vi "Main.vi"() -> ()   [LabVIEW 2017]
doc: "This Continuous Measurement sample project is based on the Queued Message Handler template.\n\nThe Event Handling Loop generates messages based on user interface actions.\n\nThe Message Handling Loop processes messages generated by the Event Handling Loop, or by other messages. There are also Acquisition and Logging message handling loop subVIs, and a chart updating loop."
uses:
  controls/UI Data.ctl
  support/libs/PMU Buffer/Buffer DATA cluster.ctl
  controls/UI State.ctl
  acquisition/Acquisition Settings.ctl
  acquisition/Acquisition State.ctl
  logging/Logging Configuration.ctl
  logging/Logging State.ctl
  support/libs/PMU Buffer/Buffer Settings.ctl
  processing/Processing Settings.ctl
  controls/Acquired Data.ctl
  <vilib>/Utility/error.llb/DialogType.ctl
  support/libs/PMU Buffer/Buffer state.ctl
  b850246f-c621-4cc8-8cdb-6c63488b8d16.vi
  d6c7b380-5ef8-42a0-a533-ce26cb609579.vi
  5953c9e4-e6ed-48ce-a3e3-f4074e595e54.vi
  308fbb3a-e3c1-4651-8528-14e79cd65b6c.vi
  e1cf4c14-b580-4597-8acf-5221adc64a8a.vi
  17f702fa-b3ef-4227-89b6-1808d4fdff79.vi
  support/Message Queue/Enqueue Message (Single).vi
  <vilib>/S3DK/PMU Recorder Light/PRL Channel Selector.vi
  support/settings/Get Config File Path.vi
  <vilib>/Utility/xml.llb/Read From XML File.vi
  <vilib>/Utility/xml.llb/Read From XML File(string).vi
  <vilib>/Utility/xml.llb/Write to XML File.vi
  <vilib>/Utility/xml.llb/Write to XML File(string).vi
  <vilib>/Utility/error.llb/Error Cluster From Error Code.vi
  <vilib>/ErrorRing/Error Ring.xnode
  acquisition/Acquisition.lvlib
  logging/Logging.lvlib
  support/User Event - Stop/User Event - Stop.lvlib
  support/Message Queue/Message Queue.lvlib
  support/settings/Settings Dialog.vi
  support/settings/Settings.lvlib
  processing/Processing.lvlib
  support/libs/PMU Buffer/PMU data buffer.lvlib
  <vilib>/S3DK/PMU Recorder Light/PMU Recorder Light.lvlib
panel:
  in  "Data Selector":bool
  in  "PRL Visible":bool
  out "Buffer Active":bool
  out "Config File":bool
  out "Connected":bool
  out "Error":bool
  out "Processing":bool=TRUE
  out "Display":bool
  out "Acquisition":bool=TRUE
  out "Events":bool=TRUE
  out "Buffer":bool
  out "UI Control":bool
  out "Waveform Chart":dbl[](graph)
  in  "Settings":bool
  in  "Start":bool
  in  "Stop":bool
  out "Status":string
  in  "Exit":bool
  # "Continuous Measurement Data Logger"
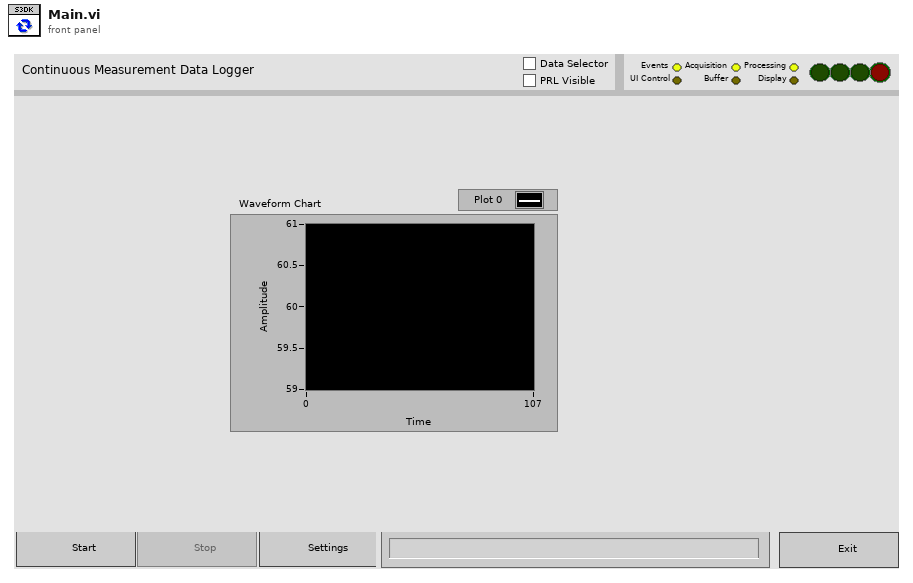
[diagram p1: front panel]
types:
  T1 = cluster{"Acq":refnum<notifier>, "Log":refnum<notifier>, "Proc":refnum<notifier>}
  T2 = typedef "Acquired Data.ctl" = cluster{"Data":dbl[]}
  T3 = typedef "Processing.lvlib/Processing Settings.ctl" = cluster{"Settings":string, "Parameters":T4, "Refresh Rate":u32}
  T4 = typedef "PMU data buffer.lvlib/Buffer Settings.ctl" = cluster{"Index":i32, "Size":i32, "Samples":i32, "Ordered ?":bool}
  T5 = typedef "Logging.lvlib/Logging Configuration.ctl" = cluster{"Logging State":T6, "Settings":string, "Buffer":T4}
  T6 = typedef "Logging.lvlib/Logging State.ctl" = enum16{"Idle", "Logging"}
  T7 = typedef "Acquisition.lvlib/Acquisition Settings.ctl" = cluster{"State":T8, "Settings":string, "Online":bool, "S3DK":cluster{"Signals":cluster{"Phasor":string[], "Analog":string[], "Digital":string[]}}, "CSV":cluster{"CSV Path":path, "Index":i32, "Parcel Length":i32, "EOF?":bool}}
  T8 = typedef "Acquisition.lvlib/Acquisition State.ctl" = enum16{"Idle", "Idle S3DK", "Acquiring S3DK", "Idle CSV", "Acquiring CSV"}
  T9 = typedef "UI State.ctl" = enum16{"Idle", "Acquiring and Logging", "Waiting for Exit", "Waiting for Exit (Acq Stopped)", "Waiting for Exit (Log Stopped)", "Waiting for Stop", "Waiting for Stop (Acq Stopped)", "Waiting for Stop (Log Stopped)"}
  T10 = typedef "PMU data buffer.lvlib/Buffer DATA cluster.ctl" = cluster{timestamp, csg[], sgl[]}
  T11 = typedef "UI Data.ctl" = cluster{"Start Ref":refnum<vi>, "Stop Ref":refnum<vi>, "Settings Ref":refnum<vi>, "Exit Ref":refnum<vi>, "Status Ref":refnum<vi>, "Data Ref":refnum<vi>, "Data Selector":refnum<vi>, "PRL Visible":refnum<vi>}
  T12 = typedef "Message Queue.lvlib/All Message Queues.ctl" = cluster{"UI":refnum<queue>, "Acquisition":refnum<queue>, "Logging":refnum<queue>, "Processing":refnum<queue>}
  T13 = enum16{"Run", "Startup", "Get Status", "Pause", "Continue", "Shutdown", "Abort", "Open Panel", "Close Panel"}
  T14 = typedef "DialogType.ctl" = u16
  T15 = enum32{"Invalid", "Standard", "Closed", "Hidden", "Minimized", "Maximized"}
  T16 = cluster{"Data Cluster":T7, "Logging Configuration":T5, "Processing Settings":T3}
  T17 = typedef "Settings.lvlib/Settings.ctl" = cluster{"Acquisition":T7, "Logging":T5, "Processing":T3}
  T18 = typedef "PMU data buffer.lvlib/Buffer state.ctl" = enum16{"Init", "Change Size", "Flush", "Exit", "Add", "Get", "Hist_Toggle", "Add_Serv"}
  T19 = typedef "PMU data buffer.lvlib/Buffer DATA OUT ordered.ctl" = cluster{"Timestamp":timestamp[], "Phasor":csg[][], "Analog":sgl[][]}
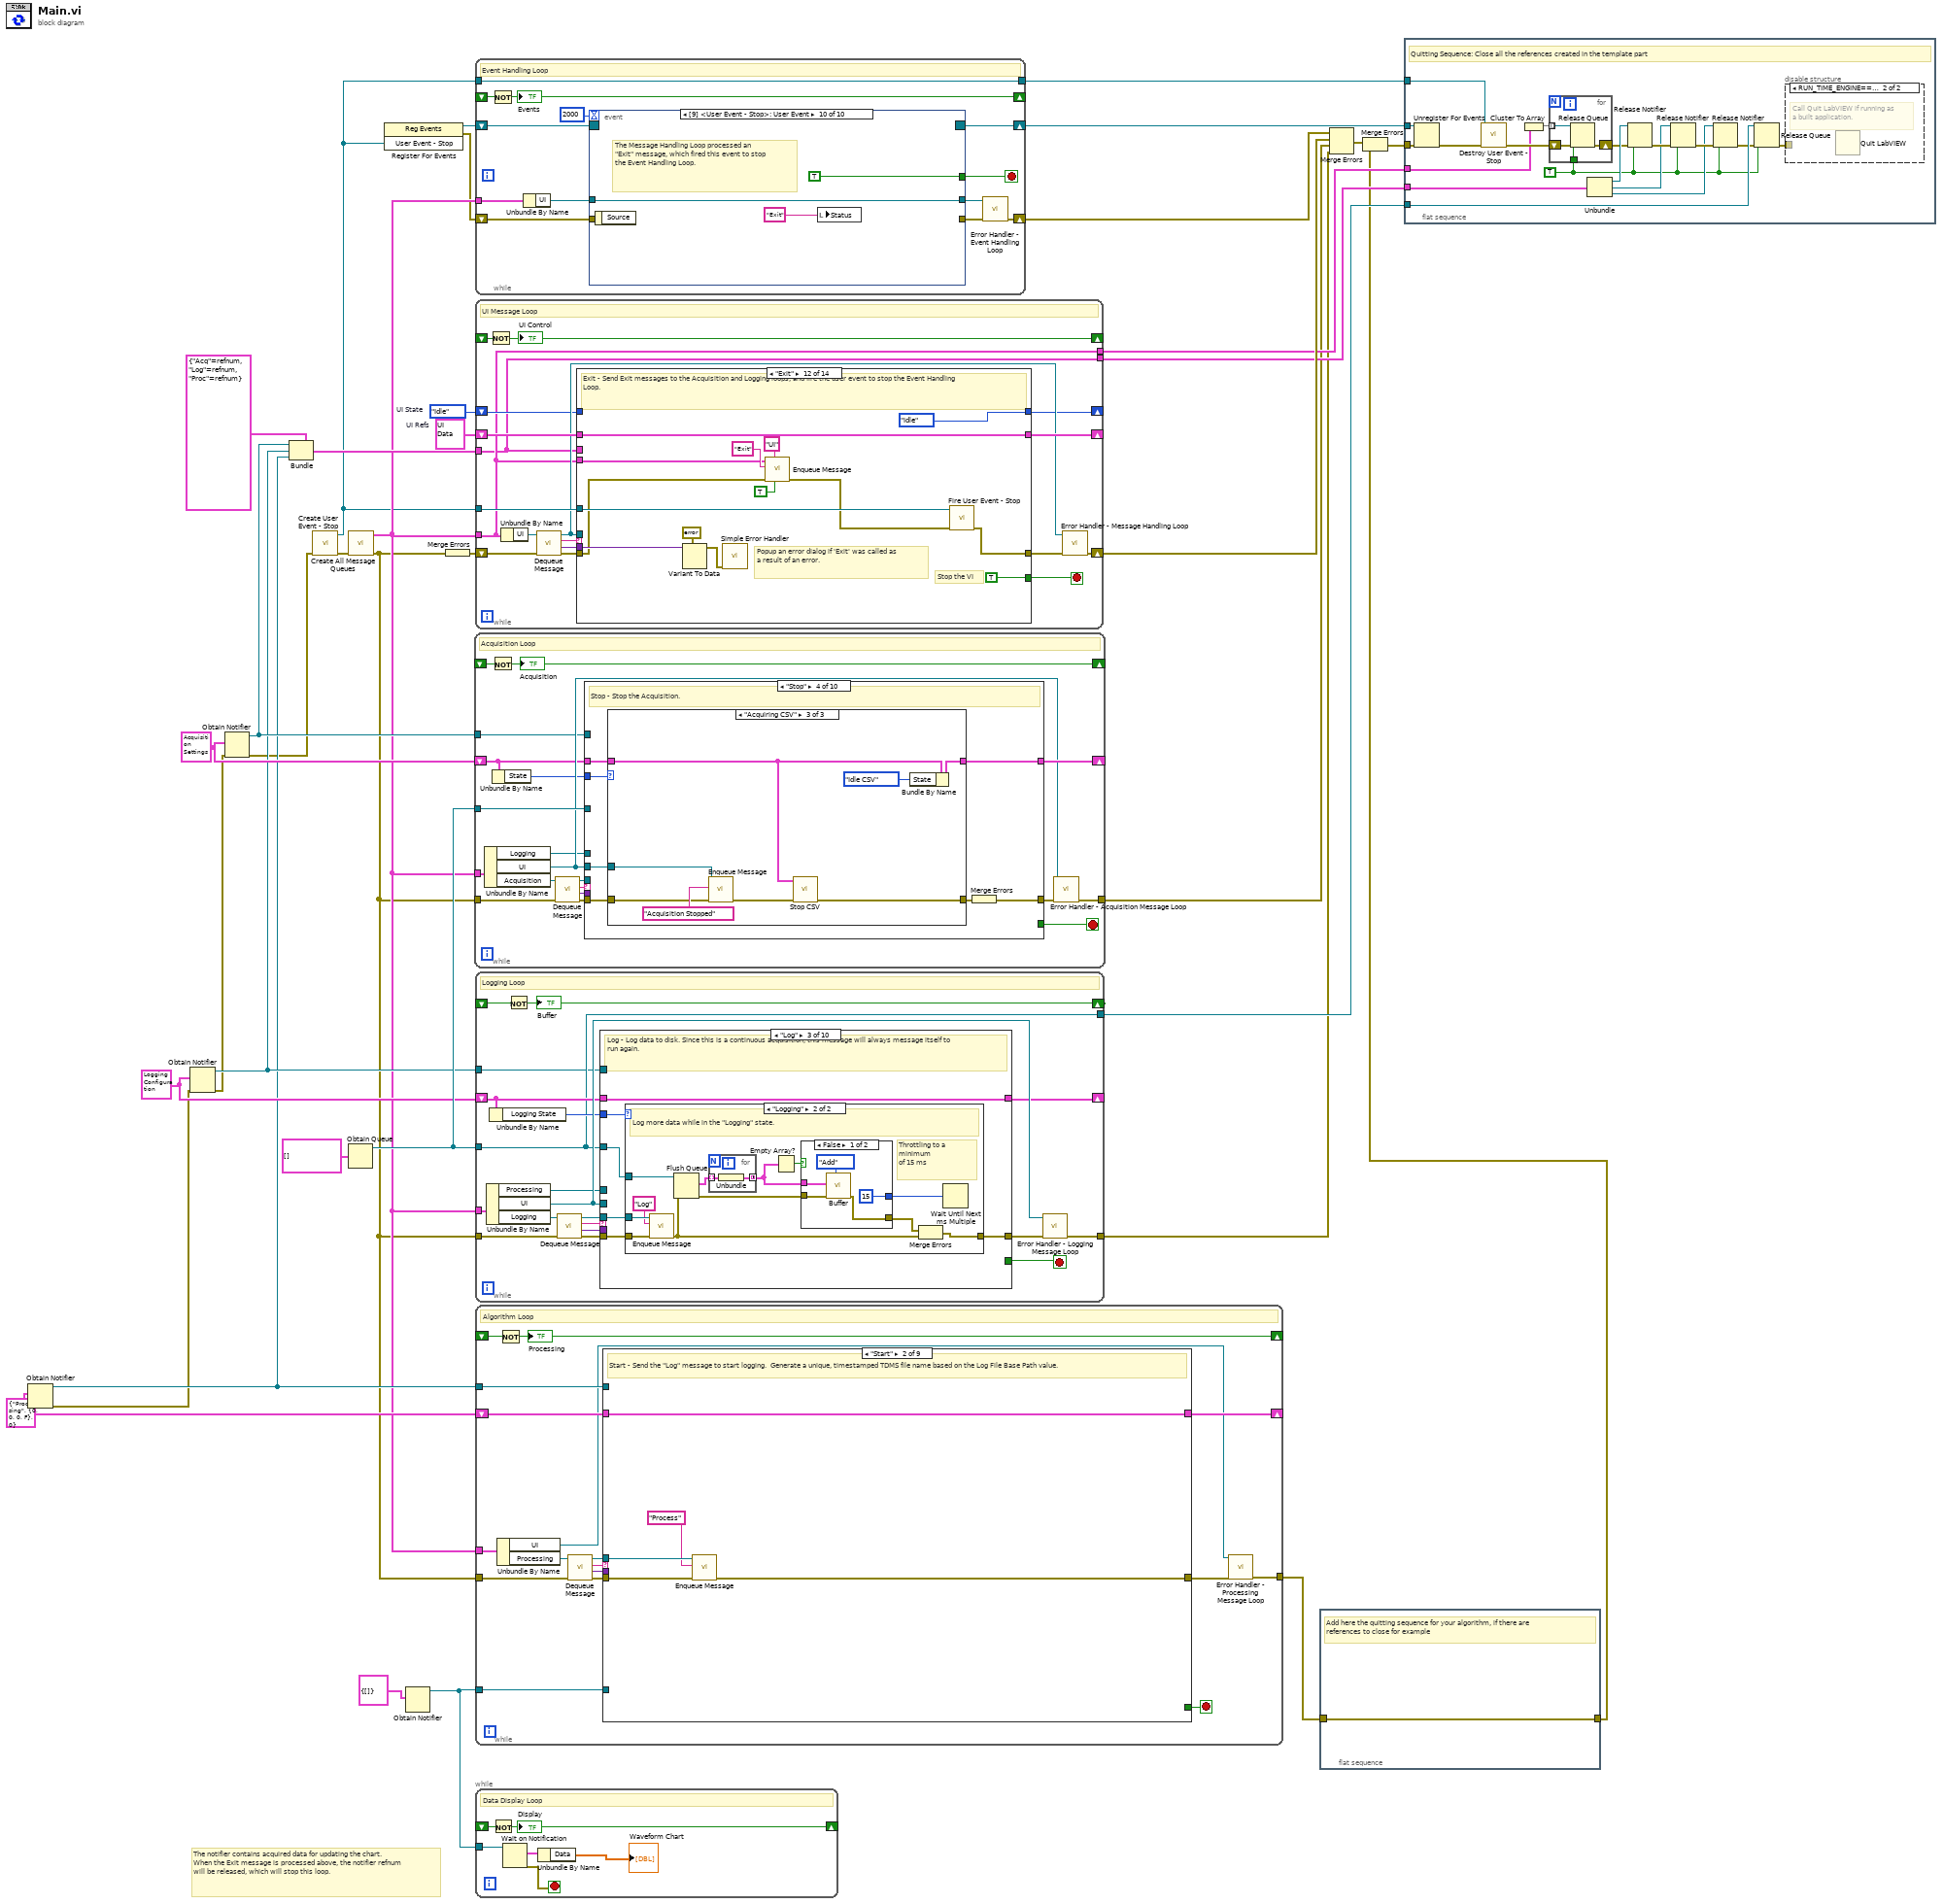
[diagram p0: block diagram]
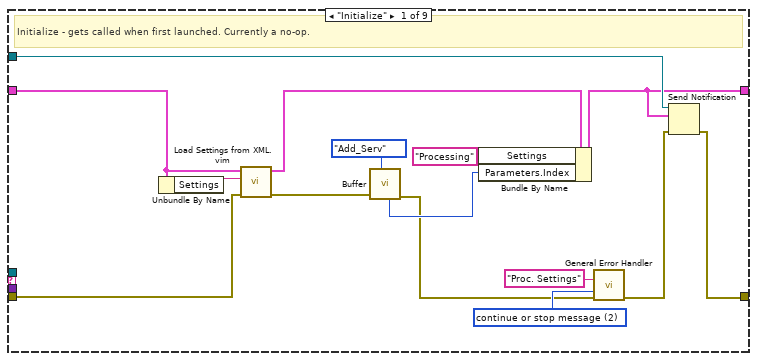
[diagram p3: hidden frame]
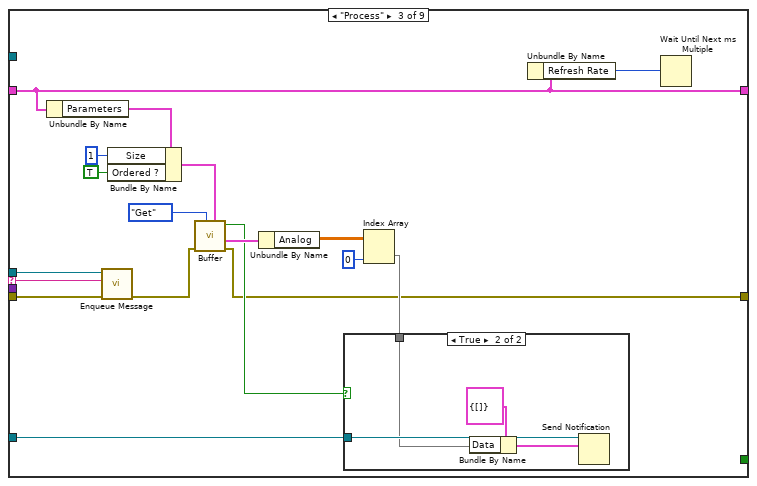
[diagram p4: hidden frame]
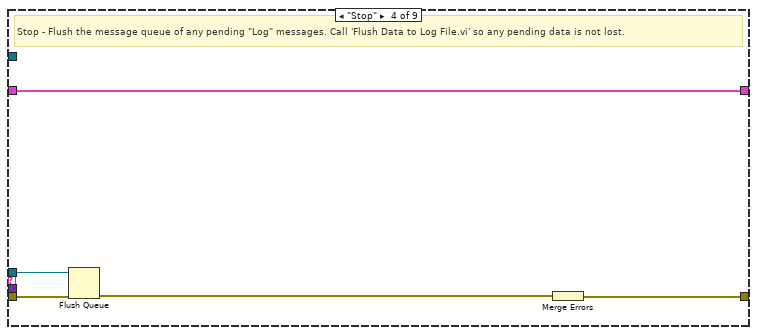
[diagram p6: hidden frame]
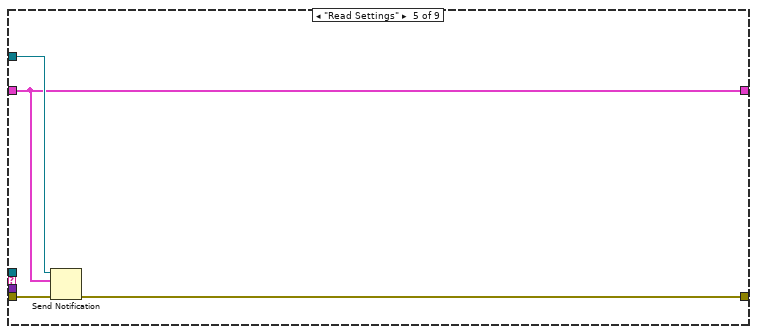
[diagram p7: hidden frame]
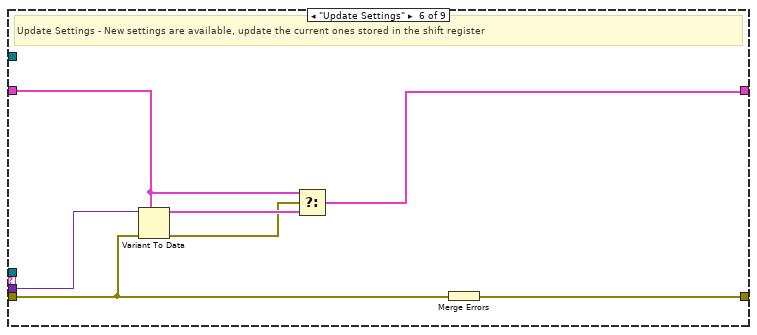
[diagram p8: hidden frame]
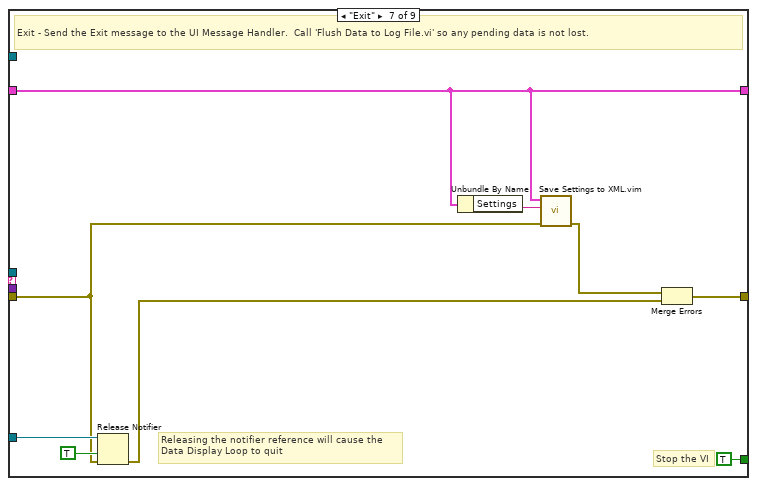
[diagram p9: hidden frame]
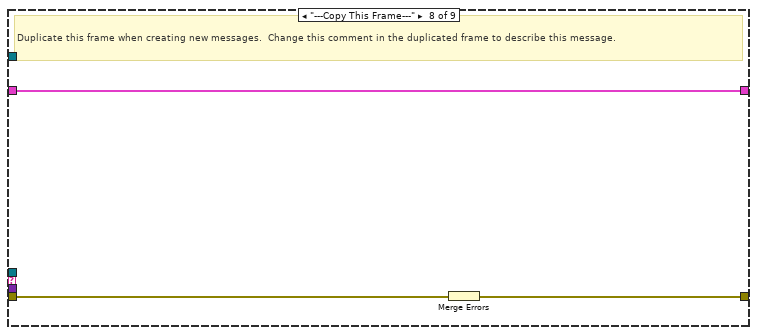
[diagram p10: hidden frame]
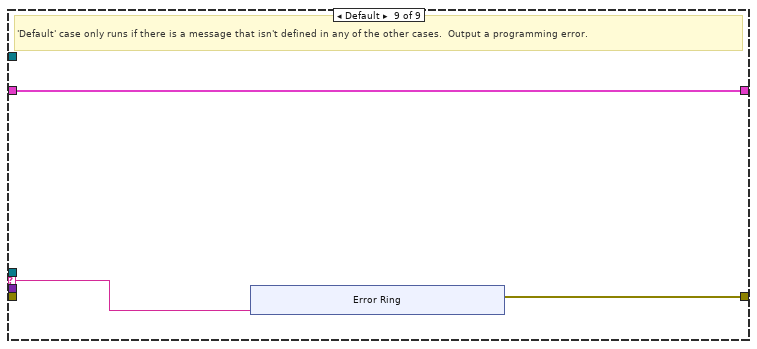
[diagram p11: hidden frame]
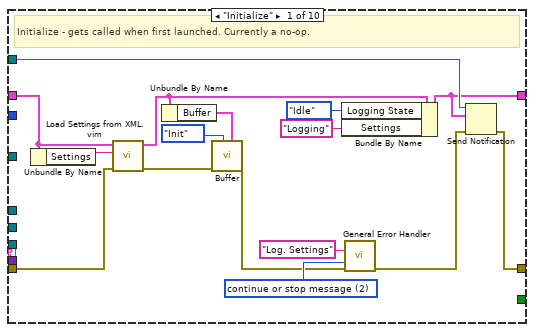
[diagram p12: hidden frame]
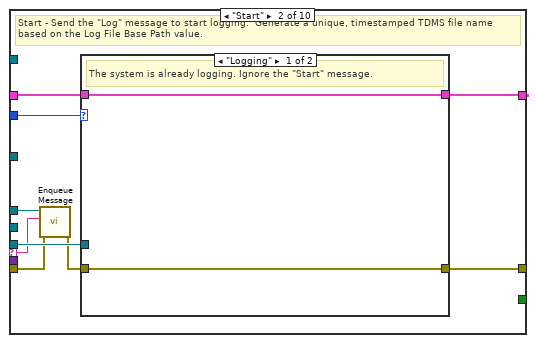
[diagram p13: hidden frame]
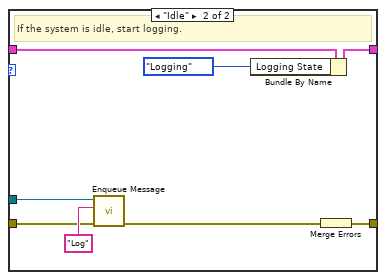
[diagram p14: hidden frame]
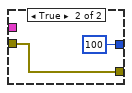
[diagram p16: hidden frame]
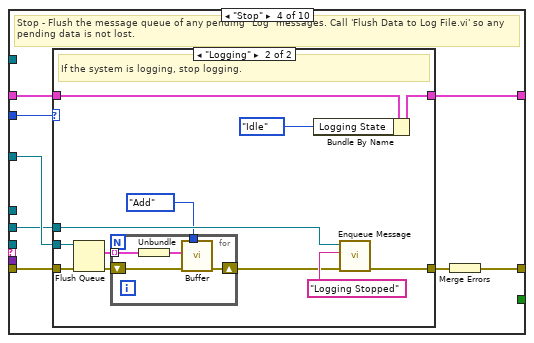
[diagram p17: hidden frame]
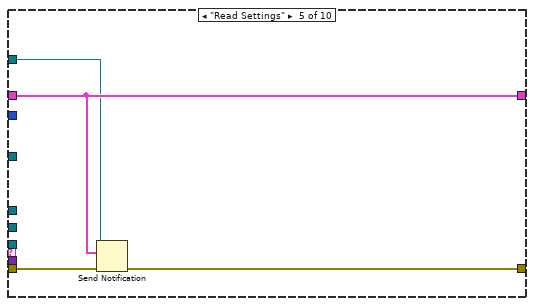
[diagram p19: hidden frame]
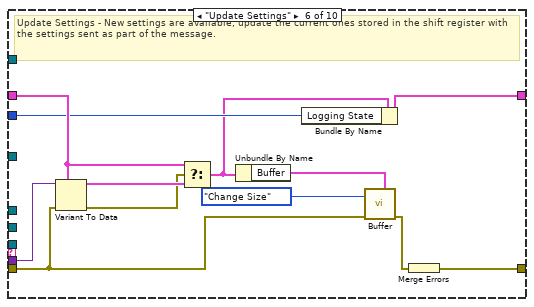
[diagram p20: hidden frame]
diagram:
  w25 = T3 {"Settings"="Processing", "Parameters"={"Index"=0, "Size"=0, "Samples"=0, "Ordered ?"=FALSE}, "Refresh Rate"=0} ("Processing Settings")
  w26 = T5 {"Logging State"=enum."Idle", "Settings"="Logging", "Buffer"={"Index"=0, "Size"=15000, "Samples"=0, "Ordered ?"=FALSE}} ("Logging Configuration")
  w27 = T7 {"State"=enum."Idle S3DK", "Settings"="Acquisition", "Online"=FALSE, "S3DK"={"Signals"={"Phasor"=[], "Analog"=[], "Digital"=[]}}, "CSV"={"CSV Path"=path "", "Index"=0, "Parcel Length"=0, "EOF?"=FALSE}} ("Data Cluster")
  w35 = UI_State."Idle"  # UI State
  w36 = T11 {"Start Ref"=refnum, "Stop Ref"=refnum, "Settings Ref"=refnum, "Exit Ref"=refnum, "Status Ref"=refnum, "Data Ref"=refnum, "Data Selector"=refnum, "PRL Visible"=refnum}  # UI Refs
  # "The notifier contains acquired data for updating the chart. When the Exit message is processed above, the notifier refnum will be released, which will stop this loop."
  n1 = Obtain Notifier(notification data type=w25) -> (notifier out=w22:refnum<notifier>, error out=w19:errorcluster)  [unwired: 3 in, 1 out]
  n2 = Obtain Notifier(notification data type=w26, error in (no error)=w19) -> (notifier out=w23:refnum<notifier>, error out=w20:errorcluster)  [unwired: 2 in, 1 out]
  n3 = Obtain Notifier(notification data type=w27, error in (no error)=w20) -> (notifier out=w24:refnum<notifier>, error out=w21:errorcluster)  [unwired: 2 in, 1 out]
  n4 = Bundle(cluster=T1 {"Acq"=refnum, "Log"=refnum, "Proc"=refnum} ("output cluster"), "Acq"=w24, "Log"=w23, "Proc"=w22) -> (w18:T1)
  n5 = call "Create User Event - Stop.vi"("error in (no error)"=w21) -> ("error out"=w37:errorcluster, "User Event - Stop"=w7:refnum<user-event>)  [unwired: 9 in]
  n6 = Obtain Queue(element data type=T10[] []) -> (queue out=w31:refnum<queue>)  [unwired: 4 in, 2 out]
  n7 = call "Create All Message Queues.vi"("error in (no error)"=w37) -> ("error out"=w12:errorcluster, "Message Queues out"=w16:T12)  [unwired: 9 in]
  n8 = register-events(w7) -> (reference out=w33:refnum<event-registration>, error out=w2:errorcluster)  [unwired: 2 in]
  n9 = Obtain Notifier(notification data type=T2 {"Data"=[]} ("Display Data")) -> (notifier out=w28:refnum<notifier>)  [unwired: 3 in, 2 out]
  n10 = Merge Errors(w12) -> (w32:errorcluster)
  n11 = while {
    shift-right: [w56] -> _
    shift-left: w27 -> [w42]
    tunnel: w31 -> [w50]
    tunnel: w16 -> [w47]
    shift-right: [w43] -> _
    shift-left: _ -> [w44]
    tunnel: w24 -> [w40]
    tunnel: w12 -> [w54]
    tunnel: [w39] -> w13
    stop <- w55 stop-if-true
    # "Acquisition Loop"
    n12 = Unbundle By Name(w47) -> ("Logging"=w38:refnum<queue>, "UI"=w46:refnum<queue>, "Acquisition"=w45:refnum<queue>)
    n13 = Not(x=w44) -> (.not. x?=w43:bool)
    "Acquisition" <- w43
    n14 = Unbundle By Name(w42) -> ("State"=w41:T8)
    n15 = call "Dequeue Message.vi"("error in (no error)"=w54, "Message Queue"=w45) -> ("error out"=w53:errorcluster, "Message Data"=w51:variant, "Message"=w52:string, "dup Message Queue"=w48:refnum<queue>)  [unwired: 6 in]
    n16 = case "Message Cases" shown="\"Stop\"" w52 {
      selector: w52 -> [_ _ w118 _ _ _ _ _ _ w263]
      tunnel: w48 -> [_ w77 w122 _ _ w184 _ _ _ _]
      tunnel: w53 -> [w67 w78 w121 w159 w182 w192 w208 w246 w262 _]
      tunnel: [w57 w79 w114 w160 w181 w196 w215 w250 w260 w264] -> w49
      tunnel: w42 -> [w66 w72 w116 w157 w180 w189 w213 w248 w261 w265]
      tunnel: [w58 w76 w115 w154 w180 w191 w212 w243 w261 w265] -> w56
      tunnel: [_ _ _ _ _ _ _ TRUE _ _] -> w55
      tunnel: w51 -> [_ _ _ _ _ w195 _ _ _ _]
      tunnel: w46 -> [_ _ w113 w155 _ _ w211 _ _ _]
      tunnel: w50 -> [_ _ w120 _ _ _ _ _ _ _]
      tunnel: w41 -> [_ w75 w119 w156 _ w190 w214 w244 _ _]
      tunnel: w40 -> [w59 _ _ _ w179 _ _ _ _ _]
      tunnel: w38 -> [_ _ _ _ _ _ w210 _ _ _]
      frame "Initialize" {
        w68 = T14 2 items=["no dialog", "OK message", "continue or stop message", "OK message + warnings", "continue/stop + warnings"] ("type of dialog (OK msg:1)")
        # "Initialize  - Initialize is currently a no-op.  The hardware initialization takes place in the 'Start' message."
        n17 = Unbundle By Name(w66) -> ("Settings"=w65:string)
        n18 = call "Load Settings from XML.vim"("error in (no error)"=w67, "Settings File Name"=w65, "Settings In"=w66) -> ("error out"=w62:errorcluster, "Settings Out"=w61:T7)  [unwired: 7 in]
        n19 = Bundle By Name(cluster=w61, "State"=Acquisition_State."Idle" ("Acquisition State"), "Settings"="Acquisition", "Online"=TRUE ("Status.Online")) -> (w58:T7)
        n20 = call <vilib>:"General Error Handler.vi"("[error source] (\" \")"="Acq. Settings" ("[error source] (\" \")"), "type of dialog (OK msg:1)"=w68, "error in (no error)"=w62) -> ("error out"=w60:errorcluster)  [unwired: 8 in, 4 out]
        n21 = Send Notification(notification=w58, notifier=w59, error in (no error)=w60) -> (error out=w57:errorcluster)  [unwired: 1 out]
      }
      frame "Start" {
        # "Start - Configure and start the acquisition."
        n22 = Unbundle By Name(w72) -> ("Online"=w71:bool)
        n23 = call-poly "Enqueue Message.vi"("error in (no error)"=w78, "Message"="Acquire", "Message Queue"=w77) -> ("error out"=w73:errorcluster)  [unwired: 7 in, 1 out]
        n24 = case shown="\"Idle\"" w75 {
          tunnel: [w83 w88 w90 w93] -> w79
          tunnel: w72 -> [w85 w89 w91 w96]
          tunnel: [w81 w87 w91 w95] -> w76
          tunnel: w73 -> [w84 w88 w90 w92]
          tunnel: w71 -> [_ _ _ w94]
          frame "Idle S3DK" {
            # "Restart the PDC streaming real time data"
            n25 = call <vilib>:"PRL Remote.vi"("error in (no error)"=w84, "Action"=T13."Continue") -> ("error out"=w83:errorcluster)  [unwired: 4 in, 5 out]
            n26 = Bundle By Name(cluster=w85, "State"=Acquisition_State."Acquiring S3DK") -> (w81:T7)
          }
          frame "Idle CSV" {
            n27 = Bundle By Name(cluster=w89, "State"=Acquisition_State."Acquiring CSV") -> (w87:T7)
          }
          frame Default {
            # "By default, ignorre the message as not in IDLE state"
          }
          frame "Idle" {
            # "If the system is idle, start the acquisition."
            n28 = case shown="True" w94 {
              tunnel: w96 -> [w98 w109]
              tunnel: [w104 w111] -> w95
              tunnel: [w99 w106] -> w93
              tunnel: w92 -> [w100 w105]
              frame False {
                n29 = call "Initialize CSV.vi"("error in (no error)"=w100, "Settings IN"=w98) -> ("error out"=w101:errorcluster, "Settings OUT"=w102:T7)  [unwired: 8 in]
                n30 = call "Configure CSV.vi"("error in (no error)"=w101, "Settings IN"=w102) -> ("error out"=w99:errorcluster, "Settings OUT"=w97:T7)  [unwired: 8 in]
                n31 = Bundle By Name(cluster=w97, "State"=Acquisition_State."Acquiring CSV") -> (w104:T7)
              }
              frame True {
                n32 = call "Initialize S3DK.vi"("error in (no error)"=w105, "Settings IN"=w109) -> ("error out"=w108:errorcluster, "Settings OUT"=w107:T7)  [unwired: 8 in]
                n33 = call "Configure S3DK.vi"("error in (no error)"=w108, "Settings IN"=w107) -> ("error out"=w106:errorcluster, "Settings OUT"=w112:T7)  [unwired: 8 in]
                n34 = Bundle By Name(cluster=w112, "State"=Acquisition_State."Acquiring S3DK" ("Acquisition State")) -> (w111:T7)
              }
            }
          }
        }
      }
      frame "Acquire" {
        # "Throttling to a min of 10 ms in the loop"
        # "Acquire - Acquire data from the hardware. Since this is a continuous acquisition, this message will always message itself to run again."
        n35 = case shown="\"Acquiring CSV\"" w119 {
          tunnel: [w126 w132 w137] -> w114
          tunnel: w122 -> [w130 _ w140]
          tunnel: w121 -> [w129 w132 w141]
          tunnel: [w123 w131 w133] -> w115
          tunnel: w116 -> [w125 w131 w143]
          tunnel: w120 -> [w124 _ w144]
          tunnel: w118 -> [w128 _ w139]
          tunnel: w113 -> [_ _ w136]
          frame "Acquiring S3DK" {
            # "Acquire more data while in the \"Acquiring\" state."
            n36 = call-poly "Enqueue Message.vi"("error in (no error)"=w129, "Message"=w128, "Message Queue"=w130) -> ("error out"=w127:errorcluster)  [unwired: 7 in, 1 out]
            n37 = call "Acquire S3DK.vi"("error in (no error)"=w127, "DATA IN"=w124, "Hardware Resources in"=w125) -> ("error out"=w126:errorcluster, "Hardware Resources out"=w123:T7)  [unwired: 7 in]
          }
          frame Default {
          }
          frame "Acquiring CSV" {
            n38 = call-poly "Enqueue Message.vi"("error in (no error)"=w141, "Message"=w139, "Message Queue"=w140) -> ("error out"=w142:errorcluster)  [unwired: 7 in, 1 out]
            n39 = call "Acquire CSV.vi"("error in (no error)"=w142, "DATA IN"=w144, "Hardware Resources in"=w143) -> ("error out"=w138:errorcluster, "Hardware Resources out"=w134:T7)  [unwired: 7 in]
            n40 = Unbundle By Name(w134) -> ("CSV.EOF?"=w135:bool)
            n41 = case shown="True" w135 {
              tunnel: w138 -> [w146 w152]
              tunnel: [w146 w151] -> w137
              tunnel: w136 -> [_ w150]
              tunnel: w134 -> [w145 w149]
              tunnel: [w145 w148] -> w133
              frame False {
              }
              frame True {
                n42 = Bundle By Name(cluster=w149, "CSV.Index"=0 ("CSV .Index (file reading)")) -> (w148:T7)
                n43 = call-poly "Enqueue Message.vi"("error in (no error)"=w152, "Message"="Stop", "Message Queue"=w150) -> ("error out"=w151:errorcluster)  [unwired: 7 in, 1 out]
              }
            }
          }
        }
        n44 = Wait Until Next ms Multiple(millisecond multiple=u32 10) -> ()  [unwired: 1 out]
      }
      frame "Stop" {
        # "Stop - Stop the Acquisition."
        n45 = case shown="\"Acquiring CSV\"" w156 {
          tunnel: w159 -> [w162 w168 w174]
          tunnel: [w162 w163 w171] -> w158
          tunnel: w157 -> [w161 w167 w173]
          tunnel: w155 -> [_ w170 w175]
          tunnel: [w161 w166 w177] -> w154
          frame Default {
            # "The system is already idle. Ignore the \"Stop\" message."
          }
          frame "Acquiring S3DK" {
            # "If the system is acquiring, stop the acquisition."
            n46 = call-poly "Enqueue Message.vi"("error in (no error)"=w168, "Message"="Acquisition Stopped", "Message Queue"=w170) -> ("error out"=w164:errorcluster)  [unwired: 7 in, 1 out]
            n47 = call "Stop S3DK.vi"("error in (no error)"=w164, "Hardware Resources in"=w167) -> ("error out"=w163:errorcluster)  [unwired: 9 in]
            n48 = Bundle By Name(cluster=w167, "State"=Acquisition_State."Idle S3DK") -> (w166:T7)
          }
          frame "Acquiring CSV" {
            n49 = call-poly "Enqueue Message.vi"("error in (no error)"=w174, "Message"="Acquisition Stopped", "Message Queue"=w175) -> ("error out"=w172:errorcluster)  [unwired: 7 in, 1 out]
            n50 = call "Stop CSV.vi"("error in (no error)"=w172, "Hardware Resources in"=w173) -> ("error out"=w171:errorcluster)  [unwired: 9 in]
            n51 = Bundle By Name(cluster=w173, "State"=Acquisition_State."Idle CSV") -> (w177:T7)
          }
        }
        n52 = Merge Errors(w158) -> (w160:errorcluster)
      }
      frame "Read Settings" {
        n53 = Send Notification(notification=w180, notifier=w179, error in (no error)=w182) -> (error out=w181:errorcluster)  [unwired: 1 out]
      }
      frame "Update Settings" {
        # "New settings are available, update the current ones stored in the shift register with the settings sent as part of the message"
        n54 = Variant To Data(error in=w192, type=w189, Variant=w195) -> (data=w193:T7, error out=w194:errorcluster)
        n55 = Unbundle By Name(w189) -> ("Online"=w188:bool)
        n56 = Select(t=w189, s=w194, f=w193) -> (s? t:f=w187:T7)
        n57 = Unbundle By Name(w187) -> ("Online"=w186:bool)
        n58 = Not Equal?(x=w188, y=w186) -> (x != y?=w183:bool)
        n59 = case shown="True" w183 {
          tunnel: w192 -> [w197 w201]
          tunnel: [w197 w200] -> w185
          tunnel: w184 -> [_ w199]
          frame False {
          }
          frame True {
            # "Launch the sequence to change source of data"
            n60 = call-poly "Enqueue Message.vi"("error in (no error)"=w201, "Message"="Toggle Online", "Message Queue"=w199) -> ("error out"=w200:errorcluster)  [unwired: 7 in, 1 out]
          }
        }
        n61 = Bundle By Name(cluster=w187, "State"=w190) -> (w191:T7)
        n62 = Merge Errors(w185) -> (w196:errorcluster)
      }
      frame "Toggle Online" {
        # "Duplicate this frame when creating new messages.  Change this comment in the duplicated frame to describe this message."
        n63 = call-poly "Enqueue Message.vi"("error in (no error)"=w208, "Message"="Flush", "Message Queue"=w210) -> ("error out"=w207:errorcluster)  [unwired: 7 in, 1 out]
        n64 = case shown="\"Idle\", Default" w214 {
          tunnel: w213 -> [w222 w231 w238]
          tunnel: [w222 w231 w238] -> w212
          tunnel: [w219 w226 w235] -> w203
          tunnel: w207 -> [w220 w230 w239]
          tunnel: w211 -> [w217 w229 w240]
          tunnel: [w216 w223 w233] -> w202
          frame "Idle", Default {
            n65 = call-poly "Enqueue Message.vi"("error in (no error)"=w220, "Message Data"="Toggle Data source" ("Message"), "Message"="Update Status", "Message Queue"=w217) -> ("error out"=w219:errorcluster, "dup Message Queue"=w216:refnum<queue>)  [unwired: 6 in]
          }
          frame "Idle S3DK", "Acquiring S3DK" {
            n66 = call-poly "Enqueue Message.vi"("error in (no error)"=w230, "Message Data"="Stopping the S3DK data acquisition" ("Ready..."), "Message"="Update Status", "Message Queue"=w229) -> ("error out"=w224:errorcluster, "dup Message Queue"=w223:refnum<queue>)  [unwired: 6 in]
            n67 = call "Stop S3DK.vi"("error in (no error)"=w224, "Hardware Resources in"=w231) -> ("error out"=w232:errorcluster)  [unwired: 9 in]
            n68 = call "Shutdown S3DK.vi"("error in (no error)"=w232, "Hardware Resources in"=w231) -> ("error out"=w225:errorcluster)  [unwired: 9 in]
            n69 = Merge Errors(w225, w224) -> (w226:errorcluster)
          }
          frame "Idle CSV", "Acquiring CSV" {
            n70 = call-poly "Enqueue Message.vi"("error in (no error)"=w239, "Message Data"="Stopping the CSV data acquisition" ("Ready..."), "Message"="Update Status", "Message Queue"=w240) -> ("error out"=w234:errorcluster, "dup Message Queue"=w233:refnum<queue>)  [unwired: 6 in]
            n71 = call "Stop CSV.vi"("error in (no error)"=w234, "Hardware Resources in"=w238) -> ("error out"=w237:errorcluster)  [unwired: 9 in]
            n72 = call "Shutdown CSV.vi"("error in (no error)"=w237, "Hardware Resources in"=w238) -> ("error out"=w236:errorcluster)  [unwired: 9 in]
            n73 = Merge Errors(w236, w234) -> (w235:errorcluster)
          }
        }
        n74 = call-poly "Enqueue Message.vi"("error in (no error)"=w203, "Message Data"="Ready..." ("Ready..."), "Message"="Update Status", "Message Queue"=w202) -> ("error out"=w204:errorcluster)  [unwired: 6 in, 1 out]
        n75 = Merge Errors(w204) -> (w215:errorcluster)
      }
      frame "Exit" {
        # "Stop the VI"
        # "Exit - Send the Exit message to the UI Message Handler."
        n76 = case shown="\"Idle CSV\", \"Acquiring CSV\"" w244 {
          tunnel: w248 -> [w252 w254 w257]
          tunnel: [w253 w255 w259] -> w247
          tunnel: w246 -> [w253 w256 w258]
          tunnel: [w252 w254 w257] -> w243
          frame "Idle", Default {
          }
          frame "Idle CSV", "Acquiring CSV" {
            n77 = call "Shutdown CSV.vi"("error in (no error)"=w256, "Hardware Resources in"=w254) -> ("error out"=w255:errorcluster)  [unwired: 9 in]
          }
          frame "Idle S3DK", "Acquiring S3DK" {
            n78 = call "Shutdown S3DK.vi"("error in (no error)"=w258, "Hardware Resources in"=w257) -> ("error out"=w259:errorcluster)  [unwired: 9 in]
          }
        }
        n79 = Unbundle By Name(w243) -> ("Settings"=w249:string)
        n80 = call "Save Settings to XML.vim"("error in (no error)"=w247, "Settings File Name"=w249, "Settings In"=w243) -> ("error out"=w245:errorcluster)  [unwired: 8 in]
        n81 = Merge Errors(w245) -> (w250:errorcluster)
      }
      frame "---Copy This Frame---" {
        # "Duplicate this frame when creating new messages.  Change this comment in the duplicated frame to describe this message."
        n82 = Merge Errors(w262) -> (w260:errorcluster)
      }
      frame Default {
        # "'Default' case only runs if there is a message that isn't defined in any of the other cases.  Output a programming error."
        n83 = xnode "Error Ring"("parameter 0"=w263) -> ("error out"=w264:errorcluster)
      }
    }
    n84 = call "Error Handler - Acquisition Message Loop.vi"("error in (no error)"=w49, "Message Queue"=w46) -> ("dup error in"=w39:errorcluster)  [unwired: 8 in, 1 out]
  }
  n85 = while {
    shift-right: [w284] -> w30
    shift-left: w33 -> [w285]
    tunnel: w16 -> [w274]
    shift-right: [w277] -> _
    shift-left: _ -> [w278]
    shift-right: [w282] -> w8
    shift-left: w2 -> [w275]
    tunnel: w7 -> [w273]
    tunnel: [w273] -> w6
    stop <- w283 stop-if-true
    # "Event Handling Loop"
    n86 = Not(x=w278) -> (.not. x?=w277:bool)
    "Events" <- w277
    n87 = Unbundle By Name(w274) -> ("UI"=w279:refnum<queue>)
    n88 = event shown="[9] <User Event - Stop>: User Event" {
      selector: w285 -> [_ _ _ _ _ _ _ _ _ _]
      dyn-events: [_ _ _ _ _ _ _ _ _ _] -> w284
      timeout: 2000 -> [_ _ _ _ _ _ _ _ _ _]
      tunnel: [_ _ _ _ _ _ _ _ _ TRUE ("Discard?")] -> w283
      tunnel: w279 -> [w287 w294 w296 w300 w305 w308 w310 w317 w322 w334]
      tunnel: [w289 w292 _ w299 w303 _ w313 w315 w323 _] -> w281
      tunnel: [w286 w291 w295 w298 w304 w308 w309 w317 w322 w334] -> w280
      tunnel: w275 -> [w290 _ _ _ _ _ _ w316 w324 _]
      event Timeout {
        n89 = event-data() -> ()  [unwired: 1 in, 1 out]
        n90 = call-poly "Enqueue Message.vi"("error in (no error)"=w290, "Message"="Update Status (Acq)", "Message Queue"=w287) -> ("error out"=w289:errorcluster, "dup Message Queue"=w286:refnum<queue>)  [unwired: 7 in]
      }
      event "Start": Value Change {
        n91 = event-data() -> ()  [unwired: 1 in, 1 out]
        n92 = call-poly "Enqueue Message.vi"("Message"="Start", "Message Queue"=w294) -> ("error out"=w292:errorcluster, "dup Message Queue"=w291:refnum<queue>)  [unwired: 8 in]
      }
      event "Settings": Value Change {
        n93 = event-data() -> ()  [unwired: 1 in, 1 out]
        n94 = call-poly "Enqueue Message.vi"("Message"="Launch Settings Dialog", "Message Queue"=w296) -> ("dup Message Queue"=w295:refnum<queue>)  [unwired: 8 in, 1 out]
      }
      event "Stop": Value Change {
        n95 = event-data() -> ()  [unwired: 1 in, 1 out]
        n96 = call-poly "Enqueue Message.vi"("Message"="Stop", "Message Queue"=w300) -> ("error out"=w299:errorcluster, "dup Message Queue"=w298:refnum<queue>)  [unwired: 8 in]
      }
      event Panel Close? {
        # "Send the 'Confirm Quit' message if the user closes the panel of the VI. Discard the event so the 'Confirm Quit' message has a chance to run."
        n97 = event-data() -> ()  [unwired: 1 in, 1 out]
        n98 = call-poly "Enqueue Message.vi"("Priority Message? (F)"=TRUE, "Message"="Confirm Quit", "Message Queue"=w305) -> ("error out"=w303:errorcluster, "dup Message Queue"=w304:refnum<queue>)  [unwired: 7 in]
        n99 = event-data("Discard?"=TRUE) -> ()  [unwired: 1 in, 1 out]
      }
      event Application Instance Close {
        n100 = event-data() -> ()  [unwired: 1 in, 1 out]
      }
      event "Exit": Value Change {
        w311 = TRUE  # Priority Message
        # "The UI Message Loop handles sending the Exit message to other loops."
        n101 = event-data() -> ()  [unwired: 1 in, 1 out]
        n102 = call-poly "Enqueue Message.vi"("Priority Message? (F)"=w311, "Message"="Exit", "Message Queue"=w310) -> ("error out"=w313:errorcluster, "dup Message Queue"=w309:refnum<queue>)  [unwired: 7 in]
      }
      event "PRL Visible": Value Change {
        n103 = event-data() -> ("NewVal"=w314:bool)  [unwired: 1 in]
        n104 = Select(t=T13."Open Panel" ("Action"), s=w314, f=T13."Close Panel" ("Action")) -> (s? t:f=w320:T13)
        n105 = call <vilib>:"PRL Remote.vi"("error in (no error)"=w316, "Action"=w320) -> ("error out"=w315:errorcluster)  [unwired: 4 in, 5 out]
      }
      event "Data Selector": Value Change {
        n106 = event-data() -> ("NewVal"=w321:bool)  [unwired: 1 in]
        n107 = vi-ref "S3DK.lvlib:PMU Recorder Light.lvlib:PRL Channel Selector.vi"() -> (w325:refnum<vi>)
        n108 = case shown="False" w321 {
          tunnel: w325 -> [w328 w333]
          tunnel: w324 -> [w327 w329]
          tunnel: [w326 w330] -> w323
          frame False {
            n109 = invoke class="VI" method="FP.Close"(reference=w328, error in=w327) -> (error out=w326:errorcluster)  [unwired: 1 in, 2 out]
          }
          frame True {
            n110 = invoke class="VI" method="FP.Open"(reference=w333, error in=w329, "Activate"=TRUE ("Activate?"), "State"=T15."Standard") -> (error out=w330:errorcluster)  [unwired: 1 in, 4 out]
          }
        }
      }
      event User Event {
        # "The Message Handling Loop processed an \"Exit\" message, which fired this event to stop the Event Handling Loop."
        n111 = event-data() -> ()  [unwired: 1 in, 1 out]
        n112 = local write "Status"("Exit" ("Exit String")) -> ()
      }
    }
    n113 = call "Error Handler - Event Handling Loop.vi"("error in (no error)"=w281, "Message Queue"=w280) -> ("dup error in"=w282:errorcluster)  [unwired: 8 in, 1 out]
  }
  n114 = while {
    tunnel: w7 -> [w353]
    shift-right: [w348] -> _
    shift-left: w36 -> [w349]
    shift-right: [w343] -> _
    shift-left: w35 -> [w344]
    tunnel: w16 -> [w338]
    tunnel: w18 -> [w337]
    shift-right: [w339] -> _
    shift-left: _ -> [w340]
    tunnel: [w338] -> w15
    tunnel: [w337] -> w14
    shift-right: [w347] -> w29
    shift-left: w32 -> [w352]
    stop <- w354 stop-if-true
    # "UI Message Loop"
    n115 = Not(x=w340) -> (.not. x?=w339:bool)
    "UI Control" <- w339
    n116 = Unbundle By Name(w338) -> ("UI"=w342:refnum<queue>)
    n117 = call "Dequeue Message.vi"("error in (no error)"=w352, "Message Queue"=w342) -> ("error out"=w341:errorcluster, "Message Data"=w350:variant, "Message"=w351:string, "dup Message Queue"=w345:refnum<queue>)  [unwired: 6 in]
    n118 = case "Message Cases" shown="\"Exit\"" w351 {
      selector: w351 -> [_ _ _ _ _ _ _ _ _ _ _ _ _ w597]
      tunnel: w345 -> [w356 _ _ _ w434 _ w456 w480 _ _ w554 _ _ _]
      tunnel: w341 -> [w357 w383 w390 w395 w433 w436 w457 w481 w507 w543 w553 w583 w595 _]
      tunnel: [w364 w383 w391 w404 w418 w451 w454 w478 w523 w546 w552 w589 w594 w596] -> w346
      tunnel: [_ _ _ _ _ _ _ _ _ _ _ TRUE _ _] -> w354
      tunnel: w350 -> [_ _ w389 _ _ _ _ _ _ w547 _ w585 _ _]
      tunnel: w353 -> [_ _ _ _ _ _ _ _ _ _ _ w590 _ _]
      tunnel: w349 -> [w361 w382 w385 w403 w430 w450 w459 w483 w525 w550 w556 w588 w593 w599]
      tunnel: [w361 w369 w385 w403 w430 w450 w459 w483 w525 w550 w556 w588 w593 w599] -> w348
      tunnel: w344 -> [_ _ w384 w402 _ w440 w458 w482 w524 w545 w555 _ w592 w598]
      tunnel: [UI_State."Idle" ("UI State") UI_State."Idle" ("UI State") w384 w402 UI_State."Acquiring and Logging" ("UI State") w441 w455 w479 w524 w545 w551 UI_State."Idle" ("UI State") w592 w598] -> w343
      tunnel: w338 -> [_ _ _ _ w413 w437 _ _ w508 _ _ w578 _ _]
      tunnel: w337 -> [_ _ _ w397 _ _ _ _ w521 _ _ _ _ _]
      frame "Initialize" {
        # "Initialize - Get configuration settings, then message the UI to initialize, and broadcast the settings to the other message loops."
        n119 = call-poly "Enqueue Message.vi"("error in (no error)"=w357, "Message"="Init UI Refs", "Message Queue"=w356) -> ("error out"=w358:errorcluster, "dup Message Queue"=w359:refnum<queue>)  [unwired: 7 in]
        n120 = call-poly "Enqueue Message.vi"("error in (no error)"=w358, "Message Data"="Ready..." ("Ready..."), "Message"="Update Status", "Message Queue"=w359) -> ("error out"=w364:errorcluster)  [unwired: 6 in, 1 out]
      }
      frame "Init UI Refs" {
        # "Enable: Start, Exit, Settings \nDisable: Stop"
        # "Init UI Refs - Store control references for UI controls.  Also enable/disable controls appropriately."
        n121 = control-ref of="Data Selector"() -> (w371:refnum<vi>)
        n122 = control-ref of="PRL Visible"() -> (w370:refnum<vi>)
        n123 = control-ref of="Start"() -> (w375:refnum<vi>)
        n124 = control-ref of="Stop"() -> (w376:refnum<vi>)
        n125 = control-ref of="Settings"() -> (w374:refnum<vi>)
        n126 = control-ref of="Exit"() -> (w373:refnum<vi>)
        n127 = control-ref of="Status"() -> (w381:refnum<vi>)
        n128 = Bundle By Name(cluster=w382, "Start Ref"=w375, "Stop Ref"=w376, "Settings Ref"=w374, "Exit Ref"=w373, "Status Ref"=w381, "Data Selector"=w371, "PRL Visible"=w370) -> (w369:T11)
        n129 = Unbundle By Name(w369) -> ("Start Ref"=w368:refnum<vi>, "Exit Ref"=w367:refnum<vi>, "Settings Ref"=w366:refnum<vi>, "Stop Ref"=w365:refnum<vi>)
        n130 = Build Array(w368, w367, w366) -> (w379:refnum<vi>[])
        n131 = Build Array(w365) -> (w378:refnum<vi>[])
        n132 = call "Set Enable State on Multiple Controls.vi"("Enable?"=TRUE, "Controls"=w379) -> ()  [unwired: 10 in]
        n133 = call "Set Enable State on Multiple Controls.vi"("Enable?"=FALSE, "Controls"=w378) -> ()  [unwired: 10 in]
      }
      frame "Update Status" {
        # "Update Status - Convert the message data to a string to display in the Status indicator."
        n134 = Variant To Data(error in=w390, type="", Variant=w389) -> (data=→"Status":string, error out=w387:errorcluster)
        n135 = Merge Errors(w387) -> (w391:errorcluster)
      }
      frame "Update Status (Acq)" {
        # "Duplicate this frame when creating new messages.  Change this comment in the duplicated frame to describe this message."
        n136 = Unbundle By Name(w397) -> ("Acq"=w396:refnum<notifier>)
        n137 = Get Notifier Status(notifier=w396, error in (no error)=w395) -> (current notification=w393:T7, error out=w394:errorcluster)  [unwired: 3 out]
        n138 = Unbundle By Name(w393) -> ("Online"=w392:bool)
        n139 = case shown="True" w392 {
          tunnel: [w409 _] -> w401
          tunnel: [w408 _] -> w400
          tunnel: [w407 _] -> w399
          tunnel: [w405 _] -> w398
          frame True {
            n140 = call <vilib>:"PRL Remote.vi"("Action"=T13."Get Status") -> ("error out"=w406:errorcluster, "Connected"=w407:bool, "Configuration File Received"=w408:bool, "Buffer Active"=w411:bool, "Queue Active"=w410:bool)  [unwired: 5 in, 1 out]
            n141 = Unbundle By Name(w406) -> ("status"=w405:bool)
            n142 = Or(x=w410, y=w411) -> (x .or. y?=w409:bool)
          }
          frame False {
          }
        }
        "Buffer Active" <- w401
        "Config File" <- w400
        "Connected" <- w399
        "Error" <- w398
        n143 = Merge Errors(w394) -> (w404:errorcluster)
      }
      frame "Start" {
        # "Message Acquisition and Logging loops to start."
        # "Enable: Stop\nDisable: Start, Exit, Settings"
        # "Start - Enable/Disable buttons appropriately for an acquisition that has started, and update status display."
        n144 = Unbundle By Name(w430) -> ("Stop Ref"=w425:refnum<vi>, "Start Ref"=w424:refnum<vi>, "Exit Ref"=w423:refnum<vi>, "Settings Ref"=w422:refnum<vi>)
        n145 = call-poly "Enqueue Message.vi"("error in (no error)"=w433, "Message Data"="Acquiring and Logging..." ("Acquiring and Logging..."), "Message"="Update Status", "Message Queue"=w434) -> ("error out"=w421:errorcluster)  [unwired: 6 in, 1 out]
        n146 = Build Array(w424, w423, w422) -> (w428:refnum<vi>[])
        n147 = Build Array(w425) -> (w427:refnum<vi>[])
        n148 = Unbundle By Name(w413) -> ("Acquisition"=w414:refnum<queue>)
        n149 = call "Set Enable State on Multiple Controls.vi"("Enable?"=TRUE, "Controls"=w427) -> ()  [unwired: 10 in]
        n150 = call "Set Enable State on Multiple Controls.vi"("Enable?"=FALSE, "Controls"=w428) -> ()  [unwired: 10 in]
        n151 = call-poly "Enqueue Message.vi"("error in (no error)"=w421, "Message"="Start", "Message Queue"=w414) -> ("error out"=w419:errorcluster)  [unwired: 7 in, 1 out]
        n152 = Unbundle By Name(w413) -> ("Logging"=w415:refnum<queue>)
        n153 = call-poly "Enqueue Message.vi"("error in (no error)"=w419, "Message"="Start", "Message Queue"=w415) -> ("error out"=w418:errorcluster)  [unwired: 7 in, 1 out]
      }
      frame "Stop" {
        # "Message Acquisition, Logging and Process loops to stop"
        # "Enable: Start, Exit, Settings\nDisable: Stop"
        # "Stop - Enable/Disable buttons appropriately for an acquisition that has stopped, and update status display."
        n154 = call-poly "Enqueue Message.vi"("Exclude"="UI", "error in (no error)"=w436, "Message"="Stop", "Message Queues in"=w437) -> ("error out"=w438:errorcluster)  [unwired: 6 in, 1 out]
        n155 = Unbundle By Name(w450) -> ("Stop Ref"=w445:refnum<vi>, "Start Ref"=w444:refnum<vi>, "Exit Ref"=w443:refnum<vi>, "Settings Ref"=w442:refnum<vi>)
        n156 = Build Array(w444, w443, w442) -> (w448:refnum<vi>[])
        n157 = Build Array(w445) -> (w447:refnum<vi>[])
        n158 = call "Set Enable State on Multiple Controls.vi"("Enable?"=FALSE, "Controls"=w447) -> ()  [unwired: 10 in]
        n159 = call "Set Enable State on Multiple Controls.vi"("Enable?"=TRUE, "Controls"=w448) -> ()  [unwired: 10 in]
        n160 = case shown="Default" w440 {
          selector: w440 -> [w452 _]
          tunnel: [w452 UI_State."Waiting for Stop" ("UI State")] -> w441
          frame "Waiting for Exit" {
          }
          frame Default {
          }
        }
        n161 = Merge Errors(w438) -> (w451:errorcluster)
      }
      frame "Acquisition Stopped" {
        # "Logic for determining what action to take when the acquisition has stopped."
        n162 = case shown="\"Waiting for Stop (Log Stopped)\"" w458 {
          selector: w458 -> [w461 _ _ _ _]
          tunnel: w457 -> [w460 w463 w465 w471 w477]
          tunnel: w456 -> [_ _ _ w469 w474]
          tunnel: [w461 UI_State."Waiting for Exit (Acq Stopped)" ("UI State") UI_State."Waiting for Stop (Acq Stopped)" ("UI State") UI_State."Idle" ("UI State") UI_State."Idle" ("UI State")] -> w455
          tunnel: [w460 w463 w465 w470 w475] -> w454
          frame Default {
          }
          frame "Waiting for Exit", "Waiting for Exit (Acq Stopped)" {
          }
          frame "Waiting for Stop", "Waiting for Stop (Acq Stopped)" {
          }
          frame "Waiting for Exit (Log Stopped)" {
            # "If we are waiting to exit, and the logging has already stopped, then the \"Acquisition Stopped\" message indicates that it is time to exit."
            n163 = call-poly "Enqueue Message.vi"("Priority Message? (F)"=TRUE, "error in (no error)"=w471, "Message"="Exit", "Message Queue"=w469) -> ("error out"=w470:errorcluster)  [unwired: 6 in, 1 out]
          }
          frame "Waiting for Stop (Log Stopped)" {
            # "If we are waiting to stop, and the logging has already stopped, then the \"Acquisition Stopped\" message indicates that it is time to stop."
            n164 = call-poly "Enqueue Message.vi"("error in (no error)"=w477, "Message Data"="Ready..." ("Ready..."), "Message"="Update Status", "Message Queue"=w474) -> ("error out"=w475:errorcluster)  [unwired: 6 in, 1 out]
          }
        }
      }
      frame "Logging Stopped" {
        # "Logic for determining what action to take when the logging has stopped."
        n165 = case shown="\"Waiting for Exit (Acq Stopped)\"" w482 {
          selector: w482 -> [w485 _ _ _ _]
          tunnel: w481 -> [w484 w487 w489 w495 w498]
          tunnel: w480 -> [_ _ _ w493 w497]
          tunnel: [w485 UI_State."Waiting for Exit (Log Stopped)" ("UI State") UI_State."Waiting for Stop (Log Stopped)" ("UI State") UI_State."Idle" ("UI State") UI_State."Idle" ("UI State")] -> w479
          tunnel: [w484 w487 w489 w494 w496] -> w478
          frame Default {
          }
          frame "Waiting for Exit", "Waiting for Exit (Log Stopped)" {
          }
          frame "Waiting for Stop", "Waiting for Stop (Log Stopped)" {
          }
          frame "Waiting for Exit (Acq Stopped)" {
            # "If we are waiting to exit, and the acquisition has already stopped, then the \"Logging Stopped\" message indicates that it is time to exit."
            n166 = call-poly "Enqueue Message.vi"("Priority Message? (F)"=TRUE, "error in (no error)"=w495, "Message"="Exit", "Message Queue"=w493) -> ("error out"=w494:errorcluster)  [unwired: 6 in, 1 out]
          }
          frame "Waiting for Stop (Acq Stopped)" {
            # "If we are waiting to stop, and the acquisition has already stopped, then the \"Logging Stopped\" message indicates that it is time to stop."
            n167 = call-poly "Enqueue Message.vi"("error in (no error)"=w498, "Message Data"="Ready..." ("Ready..."), "Message"="Update Status", "Message Queue"=w497) -> ("error out"=w496:errorcluster)  [unwired: 6 in, 1 out]
          }
        }
      }
      frame "Launch Settings Dialog" {
        w510 = 300 ("timeout in ms (-1)")
        # "Launch Settings Dialog - Launch the Settings Dialog when the user clicks the 'Settings' button."
        n168 = Unbundle(w521) -> ("Acq"=w520:refnum<notifier>, "Log"=w512:refnum<notifier>, "Proc"=w511:refnum<notifier>)
        n169 = call "Enqueue Message (same to all queues).vi"("Priority"=TRUE, "Exclude"="UI" ("y"), "error in (no error)"=w507, "Message"="Read Settings", "Message Queues in"=w508) -> ("error out"=w519:errorcluster, "Message Queues out"=w506:T12)  [unwired: 5 in]
        n170 = Wait on Notification(notifier=w520, timeout in ms (-1)=w510, error in (no error)=w519) -> (notification=w503:T7, error out=w516:errorcluster)  [unwired: 1 in, 2 out]
        n171 = Wait on Notification(notifier=w512, timeout in ms (-1)=w510, error in (no error)=w519) -> (notification=w515:T5, error out=w517:errorcluster)  [unwired: 1 in, 2 out]
        n172 = Wait on Notification(notifier=w511, timeout in ms (-1)=w510, error in (no error)=w519) -> (notification=w514:T3, error out=w518:errorcluster)  [unwired: 1 in, 2 out]
        n173 = Merge Errors(w516, w517, w518) -> (w522:errorcluster)
        n174 = Bundle("Data Cluster"=w503, "Logging Configuration"=w515, "Processing Settings"=w514) -> (w513:T16)  [unwired: 1 in]
        n175 = call-by-ref "?"("error in (no error)"=w522, "Settings in"=w513) -> ("error out"=w526:errorcluster, "Changed?"=w527:bool, "Settings out"=w509:T17)  [unwired: 8 in, 3 out]
        n176 = case shown="True" w527 {
          tunnel: w526 -> [w528 w534]
          tunnel: [w528 w533] -> w523
          tunnel: w509 -> [_ w541]
          tunnel: w506 -> [_ w530]
          frame False {
          }
          frame True {
            n177 = Unbundle(w541) -> ("Acquisition"=w540:T7, "Logging"=w539:T5, "Processing"=w538:T3)
            n178 = To Variant(anything=w540) -> (Variant=w537:variant)
            n179 = To Variant(anything=w539) -> (Variant=w536:variant)
            n180 = To Variant(anything=w538) -> (Variant=w535:variant)
            n181 = Build Array(w537, w536, w535) -> (w532:variant[])
            n182 = call "Enqueue Message (same to all queues).vi"("Exclude"="UI" ("y"), "error in (no error)"=w534, "Message Data Array"=w532, "Message"="Update Settings", "Message Queues in"=w530) -> ("error out"=w533:errorcluster)  [unwired: 5 in, 1 out]
          }
        }
      }
      frame "Error" {
        w542 = T14 2 items=["no dialog", "OK message", "continue or stop message", "OK message + warnings", "continue/stop + warnings"] ("type of dialog (OK msg:1)")
        # "Error - Display an error dialog. This message is sent by the \"Error Handler\" VIs at the end of other loops in this application."
        n183 = Variant To Data(error in=w543, type=errorcluster {"status"=FALSE, "code"=0, "source"=""} ("error constant"), Variant=w547) -> (data=w544:errorcluster, error out=w548:errorcluster)
        n184 = call <vilib>:"Simple Error Handler.vi"("type of dialog (OK msg:1)"=w542, "error in (no error)"=w544) -> ()  [unwired: 3 in, 5 out]
        n185 = Merge Errors(w548) -> (w546:errorcluster)
      }
      frame "Confirm Quit" {
        # "Confirm Quit - Message that can confirm whether or not the user wants to exit the application."
        n186 = case shown="\"Acquiring and Logging\"" w555 {
          tunnel: w554 -> [w562 w566]
          tunnel: w553 -> [w561 w565]
          tunnel: [w560 w564] -> w552
          tunnel: [UI_State."Idle" ("UI State") w563] -> w551
          frame Default {
            # "If 'Confirm Quit' comes in while the system is idle, there is no need for a confirmation message."
            n187 = call-poly "Enqueue Message.vi"("Priority Message? (F)"=TRUE, "error in (no error)"=w561, "Message"="Exit", "Message Queue"=w562) -> ("error out"=w560:errorcluster)  [unwired: 6 in, 1 out]
          }
          frame "Acquiring and Logging" {
            n188 = Two Button Dialog(message="Are you sure you want to quit while the acquisition is running?" ("Confirm Quit Message"), 1:"No" ("No"), 2:"Yes" ("Yes")) -> (T button?=w567:bool)
            n189 = case shown="False" w567 {
              tunnel: w566 -> [_ w576]
              tunnel: w565 -> [w572 w577]
              tunnel: [w572 w575] -> w564
              tunnel: [UI_State."Acquiring and Logging" ("UI State") UI_State."Waiting for Exit" ("UI State")] -> w563
              frame False {
                # "User did not want to quit."
              }
              frame True {
                n190 = call-poly "Enqueue Message.vi"("error in (no error)"=w577, "Message"="Stop", "Message Queue"=w576) -> ("error out"=w575:errorcluster)  [unwired: 7 in, 1 out]
              }
            }
          }
        }
      }
      frame "Exit" {
        # "Popup an error dialog if 'Exit' was called as a result of an error."
        # "Stop the VI"
        # "Exit - Send Exit messages to the Acquisition and Logging loops, and fire the user event to stop the Event Handling Loop."
        n191 = Variant To Data(type=errorcluster {"status"=FALSE, "code"=0, "source"=""} ("error constant"), Variant=w585) -> (data=w584:errorcluster)  [unwired: 1 in, 1 out]
        n192 = call <vilib>:"Simple Error Handler.vi"("error in (no error)"=w584) -> ()  [unwired: 4 in, 5 out]
        n193 = call-poly "Enqueue Message.vi"("Priority"=TRUE ("Priority Message? (F)"), "Exclude"="UI", "error in (no error)"=w583, "Message"="Exit", "Message Queues in"=w578) -> ("error out"=w582:errorcluster)  [unwired: 5 in, 1 out]
        n194 = call "Fire User Event - Stop.vi"("error in (no error)"=w582, "User Event - Stop"=w590) -> ("error out"=w589:errorcluster)  [unwired: 9 in]
      }
      frame "---Copy This Frame---" {
        # "Duplicate this frame when creating new messages.  Change this comment in the duplicated frame to describe this message."
        n195 = Merge Errors(w595) -> (w594:errorcluster)
      }
      frame Default {
        # "'Default' case only runs if there is a message that isn't defined in any of the other cases.  Output a programming error."
        n196 = xnode "Error Ring"("parameter 0"=w597) -> ("error out"=w596:errorcluster)
      }
    }
    n197 = call "Error Handler - Message Handling Loop.vi"("error in (no error)"=w346, "Message Queue"=w345) -> ("dup error in"=w347:errorcluster)  [unwired: 8 in, 1 out]
  }
  n198 = while {
    shift-right: [w612] -> _
    shift-left: w26 -> [w614]
    tunnel: w31 -> [w611]
    tunnel: w16 -> [w608]
    shift-right: [w615] -> _
    shift-left: _ -> [w616]
    tunnel: w23 -> [w610]
    tunnel: [w611] -> w17
    tunnel: w12 -> [w609]
    tunnel: [w620] -> w11
    stop <- w625 stop-if-true
    # "Logging Loop"
    n199 = Unbundle By Name(w608) -> ("Processing"=w607:refnum<queue>, "UI"=w617:refnum<queue>, "Logging"=w618:refnum<queue>)
    n200 = Unbundle By Name(w614) -> ("Logging State"=w613:T6)
    n201 = Not(x=w616) -> (.not. x?=w615:bool)
    "Buffer" <- w615
    n202 = call "Dequeue Message.vi"("error in (no error)"=w609, "Message Queue"=w618) -> ("error out"=w624:errorcluster, "Message Data"=w622:variant, "Message"=w623:string, "dup Message Queue"=w621:refnum<queue>)  [unwired: 6 in]
    n203 = case "Message Cases" shown="\"Log\"" w623 {
      selector: w623 -> [_ w644 _ _ _ _ _ _ _ w749]
      tunnel: w621 -> [_ w649 w665 _ _ _ _ _ _ _]
      tunnel: w624 -> [w635 w643 w663 w693 w719 w721 w738 w744 w748 _]
      tunnel: [w628 w650 w666 w696 w718 w731 w740 w743 w746 w750] -> w619
      tunnel: w614 -> [w636 w648 w662 w690 w717 w729 w735 w745 w747 w751]
      tunnel: [w626 w647 w662 w689 w717 w726 w735 w745 w747 w751] -> w612
      tunnel: [_ _ _ _ _ _ TRUE _ _ _] -> w625
      tunnel: w622 -> [_ _ _ _ _ w730 _ _ _ _]
      tunnel: w617 -> [_ _ _ w691 _ _ _ _ _ _]
      tunnel: w611 -> [_ _ w664 w694 _ _ w739 _ _ _]
      tunnel: w613 -> [_ w646 w661 w692 _ w725 _ _ _ _]
      tunnel: w610 -> [w627 _ _ _ w716 _ _ _ _ _]
      tunnel: w607 -> [_ w645 _ _ _ _ _ _ _ _]
      frame "Initialize" {
        w638 = T14 2 items=["no dialog", "OK message", "continue or stop message", "OK message + warnings", "continue/stop + warnings"] ("type of dialog (OK msg:1)")
        # "Initialize - gets called when first launched. Currently a no-op."
        n204 = Unbundle By Name(w636) -> ("Settings"=w639:string)
        n205 = call "Load Settings from XML.vim"("error in (no error)"=w635, "Settings File Name"=w639, "Settings In"=w636) -> ("error out"=w631:errorcluster, "Settings Out"=w630:T5)  [unwired: 7 in]
        n206 = Unbundle By Name(w630) -> ("Buffer"=w633:T4)
        n207 = call "Buffer.vi"("Parameters"=w633, "Mode"=Buffer_state."Init", "Error IN"=w631) -> ("Error OUT"=w632:errorcluster)  [unwired: 4 in, 4 out]
        n208 = Bundle By Name(cluster=w630, "Logging State"=Logging_State."Idle" ("State"), "Settings"="Logging") -> (w626:T5)
        n209 = call <vilib>:"General Error Handler.vi"("[error source] (\" \")"="Log. Settings" ("[error source] (\" \")"), "type of dialog (OK msg:1)"=w638, "error in (no error)"=w632) -> ("error out"=w629:errorcluster)  [unwired: 8 in, 4 out]
        n210 = Send Notification(notification=w626, notifier=w627, error in (no error)=w629) -> (error out=w628:errorcluster)  [unwired: 1 out]
      }
      frame "Start" {
        # "Start - Send the \"Log\" message to start logging.  Generate a unique, timestamped TDMS file name based on the Log File Base Path value."
        n211 = call-poly "Enqueue Message.vi"("error in (no error)"=w643, "Message"=w644, "Message Queue"=w645) -> ("error out"=w642:errorcluster)  [unwired: 7 in, 1 out]
        n212 = case shown="\"Logging\"" w646 {
          tunnel: [w651 w656] -> w650
          tunnel: w649 -> [_ w657]
          tunnel: w642 -> [w651 w655]
          tunnel: w648 -> [w652 w658]
          tunnel: [w652 w659] -> w647
          frame "Logging" {
            # "The system is already logging. Ignore the \"Start\" message."
          }
          frame "Idle" {
            # "If the system is idle, start logging."
            n213 = call-poly "Enqueue Message.vi"("error in (no error)"=w655, "Message"="Log", "Message Queue"=w657) -> ("error out"=w653:errorcluster)  [unwired: 7 in, 1 out]
            n214 = Bundle By Name(cluster=w658, "Logging State"=Logging_State."Logging" ("State")) -> (w659:T5)
            n215 = Merge Errors(w653) -> (w656:errorcluster)
          }
        }
      }
      frame "Log" {
        # "Log - Log data to disk. Since this is a continuous acquisition, this message will always message itself to run again."
        n216 = case shown="\"Logging\"" w661 {
          tunnel: [w667 w679] -> w666
          tunnel: w665 -> [_ w678]
          tunnel: w664 -> [_ w675]
          tunnel: w663 -> [w667 w676]
          frame "Idle" {
            # "Ignore \"Log\" messages when the logging is idle."
          }
          frame "Logging" {
            # "Throttling to a minimum\nof 15 ms"
            # "Log more data while in the \"Logging\" state."
            n217 = call-poly "Enqueue Message.vi"("error in (no error)"=w676, "Message"="Log", "Message Queue"=w678) -> ("error out"=w674:errorcluster)  [unwired: 7 in, 1 out]
            n218 = Flush Queue(queue=w675, error in (no error)=w674) -> (remaining elements=w669:cluster{T10[]}[], error out=w671:errorcluster)  [unwired: 1 out]
            n219 = for {
              tunnel: w669 -> [w681] mode=indexing
              tunnel: [w680] -> w668 mode=concatenating
              n220 = Unbundle(w681) -> (w680:T10[])
            }
            n221 = Empty Array?(array=w668) -> (empty?=w670:bool)
            n222 = case shown="False" w670 {
              tunnel: w671 -> [w685 w688]
              tunnel: w668 -> [w686 _]
              tunnel: [w683 w688] -> w673
              tunnel: [u32 15 ("millisecond multiple") u32 100 ("millisecond multiple")] -> w672
              frame False {
                n223 = call "Buffer.vi"("Mode"=Buffer_state."Add", "Error IN"=w685, "DATA IN"=w686) -> ("Error OUT"=w683:errorcluster)  [unwired: 4 in, 4 out]
              }
              frame True {
              }
            }
            n224 = Merge Errors(w673, w674) -> (w679:errorcluster)
            n225 = Wait Until Next ms Multiple(millisecond multiple=w672) -> ()  [unwired: 1 out]
          }
        }
      }
      frame "Stop" {
        # "Stop - Flush the message queue of any pending \"Log\" messages. Call 'Flush Data to Log File.vi' so any pending data is not lost."
        n226 = case shown="\"Logging\"" w692 {
          tunnel: [w698 w710] -> w695
          tunnel: w694 -> [_ w703]
          tunnel: w693 -> [w698 w704]
          tunnel: w691 -> [_ w709]
          tunnel: w690 -> [w697 w705]
          tunnel: [w697 w707] -> w689
          frame "Idle" {
            # "The system is already idle. Ignore the \"Stop\"."
          }
          frame "Logging" {
            # "If the system is logging, stop logging."
            n227 = Flush Queue(queue=w703, error in (no error)=w704) -> (remaining elements=w702:cluster{T10[]}[], error out=w701:errorcluster)  [unwired: 1 out]
            n228 = for {
              tunnel: w702 -> [w715] mode=indexing
              shift-right: [w713] -> w699
              shift-left: w701 -> [w712]
              tunnel: Buffer_state."Add" ("Mode") -> [w711]
              n229 = Unbundle(w715) -> (w714:T10[])
              n230 = call "Buffer.vi"("Mode"=w711, "Error IN"=w712, "DATA IN"=w714) -> ("Error OUT"=w713:errorcluster)  [unwired: 4 in, 4 out]
            }
            n231 = Bundle By Name(cluster=w705, "Logging State"=Logging_State."Idle" ("State")) -> (w707:T5)
            n232 = call-poly "Enqueue Message.vi"("error in (no error)"=w699, "Message"="Logging Stopped", "Message Queue"=w709) -> ("error out"=w710:errorcluster)  [unwired: 7 in, 1 out]
          }
        }
        n233 = Merge Errors(w695) -> (w696:errorcluster)
      }
      frame "Read Settings" {
        n234 = Send Notification(notification=w717, notifier=w716, error in (no error)=w719) -> (error out=w718:errorcluster)  [unwired: 1 out]
      }
      frame "Update Settings" {
        # "Update Settings - New settings are available, update the current ones stored in the shift register with the settings sent as part of the message."
        n235 = Variant To Data(error in=w721, type=w729, Variant=w730) -> (data=w728:T5, error out=w727:errorcluster)
        n236 = Select(t=w729, s=w727, f=w728) -> (s? t:f=w724:T5)
        n237 = Unbundle By Name(w724) -> ("Buffer"=w723:T4)
        n238 = Bundle By Name(cluster=w724, "Logging State"=w725) -> (w726:T5)
        n239 = call "Buffer.vi"("Parameters"=w723, "Mode"=Buffer_state."Change Size", "Error IN"=w721) -> ("Error OUT"=w720:errorcluster)  [unwired: 4 in, 4 out]
        n240 = Merge Errors(w720) -> (w731:errorcluster)
      }
      frame "Exit" {
        # "Stop the VI"
        # "Exit - Send the Exit message to the UI Message Handler.  Call 'Flush Data to Log File.vi' so any pending data is not lost."
        n241 = Flush Queue(queue=w739, error in (no error)=w738) -> (error out=w737:errorcluster)  [unwired: 2 out]
        n242 = call "Buffer.vi"("Mode"=Buffer_state."Exit", "Error IN"=w737) -> ("Error OUT"=w733:errorcluster)  [unwired: 5 in, 4 out]
        n243 = Unbundle By Name(w735) -> ("Settings"=w734:string)
        n244 = call "Save Settings to XML.vim"("error in (no error)"=w733, "Settings File Name"=w734, "Settings In"=w735) -> ("error out"=w732:errorcluster)  [unwired: 8 in]
        n245 = Merge Errors(w732, w738) -> (w740:errorcluster)
      }
      frame "Flush" {
        n246 = call "Buffer.vi"("Mode"=Buffer_state."Flush", "Error IN"=w744) -> ("Error OUT"=w743:errorcluster)  [unwired: 5 in, 4 out]
      }
      frame "---Copy This Frame---" {
        # "Duplicate this frame when creating new messages.  Change this comment in the duplicated frame to describe this message."
        n247 = Merge Errors(w748) -> (w746:errorcluster)
      }
      frame Default {
        # "'Default' case only runs if there is a message that isn't defined in any of the other cases.  Output a programming error."
        n248 = xnode "Error Ring"("parameter 0"=w749) -> ("error out"=w750:errorcluster)
      }
    }
    n249 = call "Error Handler - Logging Message Loop.vi"("error in (no error)"=w619, "Message Queue"=w617) -> ("dup error in"=w620:errorcluster)  [unwired: 8 in, 1 out]
  }
  n250 = while {
    tunnel: w28 -> [w763]
    shift-right: [w775] -> _
    shift-left: _ -> [w774]
    tunnel: w22 -> [w762]
    shift-right: [w765] -> _
    shift-left: w25 -> [w766]
    tunnel: w16 -> [w772]
    tunnel: w12 -> [w771]
    tunnel: [w760] -> w5
    stop <- w764 stop-if-true
    # "Algorithm Loop"
    n251 = Unbundle By Name(w772) -> ("UI"=w759:refnum<queue>, "Processing"=w773:refnum<queue>)
    n252 = Not(x=w774) -> (.not. x?=w775:bool)
    "Processing" <- w775
    n253 = call "Dequeue Message.vi"("error in (no error)"=w771, "Message Queue"=w773) -> ("error out"=w768:errorcluster, "Message Data"=w767:variant, "Message"=w769:string, "dup Message Queue"=w770:refnum<queue>)  [unwired: 6 in]
    n254 = case "Message Cases" shown="\"Start\"" w769 {
      selector: w769 -> [_ _ w812 _ _ _ _ _ w847]
      tunnel: w770 -> [_ w792 w811 w819 _ _ _ _ _]
      tunnel: w768 -> [w785 w794 w813 w820 w826 w829 w834 w845 _]
      tunnel: w766 -> [w786 w795 w797 w822 w823 w832 w836 w844 w848]
      tunnel: [w776 w795 w797 w822 w823 w828 w836 w844 w848] -> w765
      tunnel: [_ _ _ _ _ _ TRUE _ _] -> w764
      tunnel: w767 -> [_ _ _ _ _ w833 _ _ _]
      tunnel: [w778 w793 w798 w821 w825 w827 w841 w843 w846] -> w761
      tunnel: w763 -> [_ _ w803 _ _ _ w840 _ _]
      tunnel: w762 -> [w777 _ _ _ w824 _ _ _ _]
      frame "Initialize" {
        w788 = T14 2 items=["no dialog", "OK message", "continue or stop message", "OK message + warnings", "continue/stop + warnings"] ("type of dialog (OK msg:1)")
        # "Initialize - gets called when first launched. Currently a no-op."
        n255 = Unbundle By Name(w786) -> ("Settings"=w789:string)
        n256 = call "Load Settings from XML.vim"("error in (no error)"=w785, "Settings File Name"=w789, "Settings In"=w786) -> ("error out"=w780:errorcluster, "Settings Out"=w781:T3)  [unwired: 7 in]
        n257 = call "Buffer.vi"("Mode"=Buffer_state."Add_Serv", "Error IN"=w780) -> ("Error OUT"=w782:errorcluster, "Index"=w784:i32)  [unwired: 5 in, 3 out]
        n258 = Bundle By Name(cluster=w781, "Settings"="Processing", "Parameters.Index"=w784) -> (w776:T3)
        n259 = call <vilib>:"General Error Handler.vi"("[error source] (\" \")"="Proc. Settings" ("[error source] (\" \")"), "type of dialog (OK msg:1)"=w788, "error in (no error)"=w782) -> ("error out"=w779:errorcluster)  [unwired: 8 in, 4 out]
        n260 = Send Notification(notification=w776, notifier=w777, error in (no error)=w779) -> (error out=w778:errorcluster)  [unwired: 1 out]
      }
      frame "Start" {
        # "Start - Send the \"Log\" message to start logging.  Generate a unique, timestamped TDMS file name based on the Log File Base Path value."
        n261 = call-poly "Enqueue Message.vi"("error in (no error)"=w794, "Message"="Process", "Message Queue"=w792) -> ("error out"=w793:errorcluster)  [unwired: 7 in, 1 out]
      }
      frame "Process" {
        n262 = Unbundle By Name(w797) -> ("Parameters"=w808:T4)
        n263 = call-poly "Enqueue Message.vi"("error in (no error)"=w813, "Message"=w812, "Message Queue"=w811) -> ("error out"=w810:errorcluster)  [unwired: 7 in, 1 out]
        n264 = Bundle By Name(cluster=w808, "Size"=1, "Ordered ?"=TRUE) -> (w807:T4)
        n265 = call "Buffer.vi"("Parameters"=w807, "Mode"=Buffer_state."Get", "Error IN"=w810) -> ("Error OUT"=w798:errorcluster, "Output"=w804:T19, "New Element ?"=w799:bool)  [unwired: 4 in, 2 out]
        n266 = Unbundle By Name(w804) -> ("Analog"=w802:sgl[][])
        n267 = Index Array(array=w802, index (col)=0 ("disabled index (col)")) -> (element=w800:sgl[])  [unwired: 1 in]
        n268 = case shown="True" w799 {
          tunnel: w803 -> [_ w817]
          tunnel: w800 -> [_ w815]
          frame False {
          }
          frame True {
            n269 = Bundle By Name(cluster=T2 {"Data"=[]} ("Display Data"), "Data"=w815) -> (w816:T2)
            n270 = Send Notification(notification=w816, notifier=w817) -> ()  [unwired: 1 in, 2 out]
          }
        }
        n271 = Unbundle By Name(w797) -> ("Refresh Rate"=w796:u32)
        n272 = Wait Until Next ms Multiple(millisecond multiple=w796) -> ()  [unwired: 1 out]
      }
      frame "Stop" {
        # "Stop - Flush the message queue of any pending \"Log\" messages. Call 'Flush Data to Log File.vi' so any pending data is not lost."
        n273 = Flush Queue(queue=w819, error in (no error)=w820) -> (error out=w818:errorcluster)  [unwired: 2 out]
        n274 = Merge Errors(w818) -> (w821:errorcluster)
      }
      frame "Read Settings" {
        n275 = Send Notification(notification=w823, notifier=w824, error in (no error)=w826) -> (error out=w825:errorcluster)  [unwired: 1 out]
      }
      frame "Update Settings" {
        # "Update Settings - New settings are available, update the current ones stored in the shift register"
        n276 = Variant To Data(error in=w829, type=w832, Variant=w833) -> (data=w831:T3, error out=w830:errorcluster)
        n277 = Select(t=w832, s=w830, f=w831) -> (s? t:f=w828:T3)
        n278 = Merge Errors(w829) -> (w827:errorcluster)
      }
      frame "Exit" {
        # "Releasing the notifier reference will cause the \nData Display Loop to quit"
        # "Stop the VI"
        # "Exit - Send the Exit message to the UI Message Handler.  Call 'Flush Data to Log File.vi' so any pending data is not lost."
        n279 = Release Notifier(notifier=w840, force destroy? (F)=TRUE, error in (no error)=w834) -> (error out=w839:errorcluster)  [unwired: 2 out]
        n280 = Unbundle By Name(w836) -> ("Settings"=w837:string)
        n281 = call "Save Settings to XML.vim"("error in (no error)"=w834, "Settings File Name"=w837, "Settings In"=w836) -> ("error out"=w835:errorcluster)  [unwired: 8 in]
        n282 = Merge Errors(w835, w839) -> (w841:errorcluster)
      }
      frame "---Copy This Frame---" {
        # "Duplicate this frame when creating new messages.  Change this comment in the duplicated frame to describe this message."
        n283 = Merge Errors(w845) -> (w843:errorcluster)
      }
      frame Default {
        # "'Default' case only runs if there is a message that isn't defined in any of the other cases.  Output a programming error."
        n284 = xnode "Error Ring"("parameter 0"=w847) -> ("error out"=w846:errorcluster)
      }
    }
    n285 = call "Error Handler - Processing Message Loop.vi"("error in (no error)"=w761, "Message Queue"=w759) -> ("dup error in"=w760:errorcluster)  [unwired: 8 in, 1 out]
  }
  n286 = while "Data Display Loop" {
    tunnel: w28 -> [w861]
    shift-right: [w859] -> _
    shift-left: _ -> [w858]
    stop <- w860 stop-if-true
    # "Data Display Loop"
    n287 = Not(x=w858) -> (.not. x?=w859:bool)
    "Display" <- w859
    n288 = Wait on Notification(notifier=w861) -> (notification=w857:T2, error out=w860:errorcluster)  [unwired: 3 in, 2 out]
    n289 = Unbundle By Name(w857) -> ("Data"=→"Waveform Chart":dbl[])
  }
  n290 = flat-sequence {
    tunnel: w5 -> [w862]
    tunnel: [w862] -> w3
    frame #0 {
      # "Add here the quitting sequence for your algorithm, if there are references to close for example"
    }
  }
  n291 = Merge Errors(w8, w29, w13, w11) -> (w9:errorcluster)
  n292 = Merge Errors(w9, w3) -> (w4:errorcluster)
  n293 = flat-sequence {
    tunnel: w30 -> [w880]
    tunnel: w17 -> [w877]
    tunnel: w15 -> [w876]
    tunnel: w14 -> [w872]
    tunnel: w4 -> [w865]
    tunnel: w6 -> [w863]
    frame #0 {
      w866 = TRUE ("force destroy? (F)")
      # "Quitting Sequence: Close all the references created in the template part"
      n294 = Unregister For Events(event registration refnum=w880, error in=w865) -> (error out=w864:errorcluster)
      n295 = call "Destroy User Event - Stop.vi"("error in (no error)"=w864, "User Event - Stop"=w863) -> ("error out"=w878:errorcluster)  [unwired: 9 in]
      n296 = Cluster To Array(cluster=w876) -> (array=w879:refnum<queue>[])
      n297 = for {
        shift-right: [w884] -> w867
        shift-left: w878 -> [w883]
        tunnel: w866 -> [w882]
        tunnel: w879 -> [w881] mode=indexing
        n298 = Release Queue(queue=w881, force destroy? (F)=w882, error in (no error)=w883) -> (error out=w884:errorcluster)  [unwired: 2 out]
      }
      n299 = Unbundle(w872) -> ("Acq"=w871:refnum<notifier>, "Log"=w870:refnum<notifier>, "Proc"=w869:refnum<notifier>)
      n300 = Release Notifier(notifier=w871, force destroy? (F)=w866, error in (no error)=w867) -> (error out=w874:errorcluster)  [unwired: 2 out]
      n301 = Release Notifier(notifier=w870, force destroy? (F)=w866, error in (no error)=w874) -> (error out=w873:errorcluster)  [unwired: 2 out]
      n302 = Release Notifier(notifier=w869, force destroy? (F)=w866, error in (no error)=w873) -> (error out=w868:errorcluster)  [unwired: 2 out]
      n303 = Release Queue(queue=w877, force destroy? (F)=w866, error in (no error)=w868) -> (error out=w875:errorcluster)  [unwired: 2 out]
      n304 = disable-structure shown="RUN_TIME_ENGINE==True" {
        disable-tunnel: w875 -> [_ _]
        frame condition #0 (active) {
        }
        frame condition #1 {
          # "Call Quit LabVIEW if running as a built application."
          n305 = Quit LabVIEW() -> ()  [unwired: 1 in]
        }
      }
    }
  }
